vi "Write Eye Params.vi"(8 "error in (no error)":errorcluster, 10 "Eye Params":dbl[](array[numeric]), 11 "TrialBasedExperiment in":refnum<class "TrialBasedExperiment.lvclass">) -> (0 "error out":errorcluster, 3 "TrialBasedExperiment out":refnum<class "TrialBasedExperiment.lvclass">)   [LabVIEW 2011, in "TrialBasedExperiment.lvclass"]
uses:
  TrialBasedExperiment.lvclass
  TrialBasedExperiment.lvclass/TrialBasedExperiment.ctl
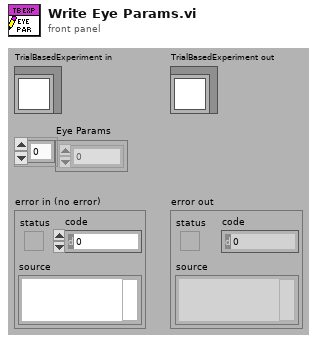
[diagram p1: front panel]
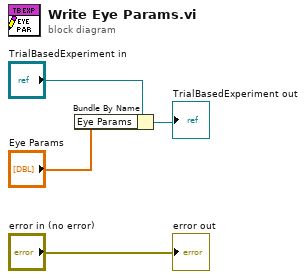
[diagram p0: block diagram]
diagram:
  n1 = Bundle By Name(cluster="TrialBasedExperiment in", "Eye Params"="Eye Params") -> (→"TrialBasedExperiment out":refnum<class "TrialBasedExperiment.lvclass">)
  "error out" <- "error in (no error)"
